vi "Length Of Demo.vi"(11 "error in":errorcluster) -> (4 "array length":i32, 6 "string length":i32, 15 "error out":errorcluster)   [LabVIEW 2026]
doc: "Calls Length Of.vim with an array and with a string, so each call site selects a different frame of the Type Specialization Structure."
uses:
  84734245-ba05-4634-a06b-5c50513cf8e7.vi
  8017acbf-eb8f-416c-95f3-1f12d461f7aa.vi
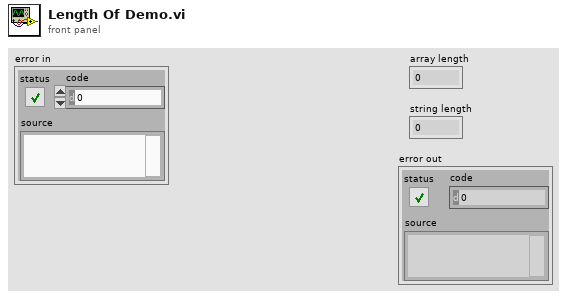
[diagram p1: front panel]
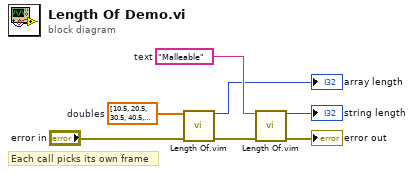
[diagram p0: block diagram]
diagram:
  w5 = "Malleable"  # text
  w7 = dbl[] [10.5, 20.5, 30.5, 40.5, 50.5, 60.5, 70.5]  # doubles
  # "Each call picks its own frame"
  n1 = call "Length Of.vim"("value in"=w7, "error in"="error in") -> ("length"=→"array length":i32, "error out"=w4:errorcluster)  [unwired: 12 in]
  n2 = call "Length Of.vim"("value in"=w5, "error in"=w4) -> ("length"=→"string length":i32, "error out"=→"error out":errorcluster)  [unwired: 12 in]
